vi "Initialize.vi"(7 "Serial Configuration":T1={"Baud Rate"=9600, "Parity"=0, "Data Bits"=7, "Stop Bits"=10, "Flow Control"=0} {"Flow Control" items=["None", "XON/XOFF", "RTS/CTS", "XON/XOFF & RTS/CTS", "DTR/DSR", "XON/XOFF & DTR/DSR"]; "Stop Bits" items=["1.0"=10, "1.5"=15, "2.0"=20]; "Data Bits" items=["7"=7, "8"=8]; "Parity" items=["None", "Odd", "Even", "Mark", "Space"]; "Baud Rate" items=["300"=300, "600"=600, "1200"=1200, "2400"=2400, "4800"=4800, "9600"=9600, "19200"=19200]}, 8 "error in (no error)":errorcluster, 9 "Reset (True)":bool=TRUE, 10 "ID Query (True)":bool=TRUE, 11 "VISA resource name":refnum<visa-resource-name>) -> (0 "error out":errorcluster, 3 "VISA resource name out":refnum<visa-resource-name>)   [LabVIEW 2019]
doc: "Establishes communication with the instrument and optionally performs an instrument identification query and/or an instrument reset. It also places the instrument in a default state needed for other instrument driver operations. Therefore, call this VI before calling other instrument driver VIs for this instrument. Generally, you need to call the <b>Initialize</b> VI only once at the beginning of an application."
uses:
  <instrlib>/Faulhaber RS232/Faulhaber RS232.lvlib
panel:
  # "(c) 2014 <Enter Company Name Here>.  ALL RIGHTS RESERVED."
  # "EDIT: Change control description to remove example text for buses not supported."
  # "EDIT: Serial settings must match those on the physical instrument.  Review user's manual to determine the correct Flow Control protocol for the instrument.  \"None\" is the least robust option for this setting, and could lead to unreliable data transmission."
  # "EDIT: If your instrument does not support ID query or Reset, remove the ID Query or Reset control from the front panel and delete the case structure with the ID Query or Reset code from the block diagram."
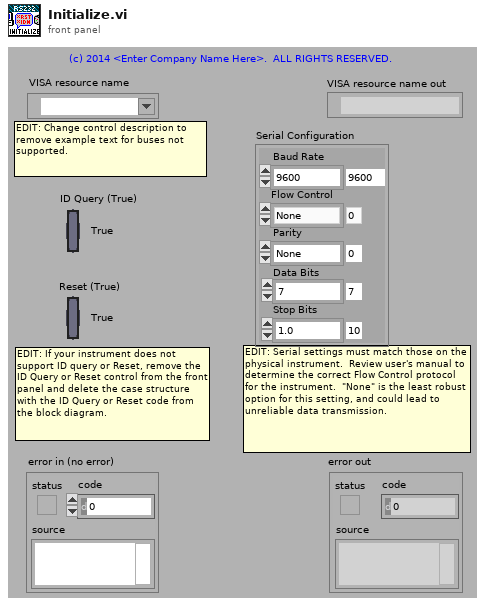
[diagram p1: front panel]
types:
  T1 = cluster{"Baud Rate":u32, "Parity":u16, "Data Bits":u16, "Stop Bits":u16, "Flow Control":u16}
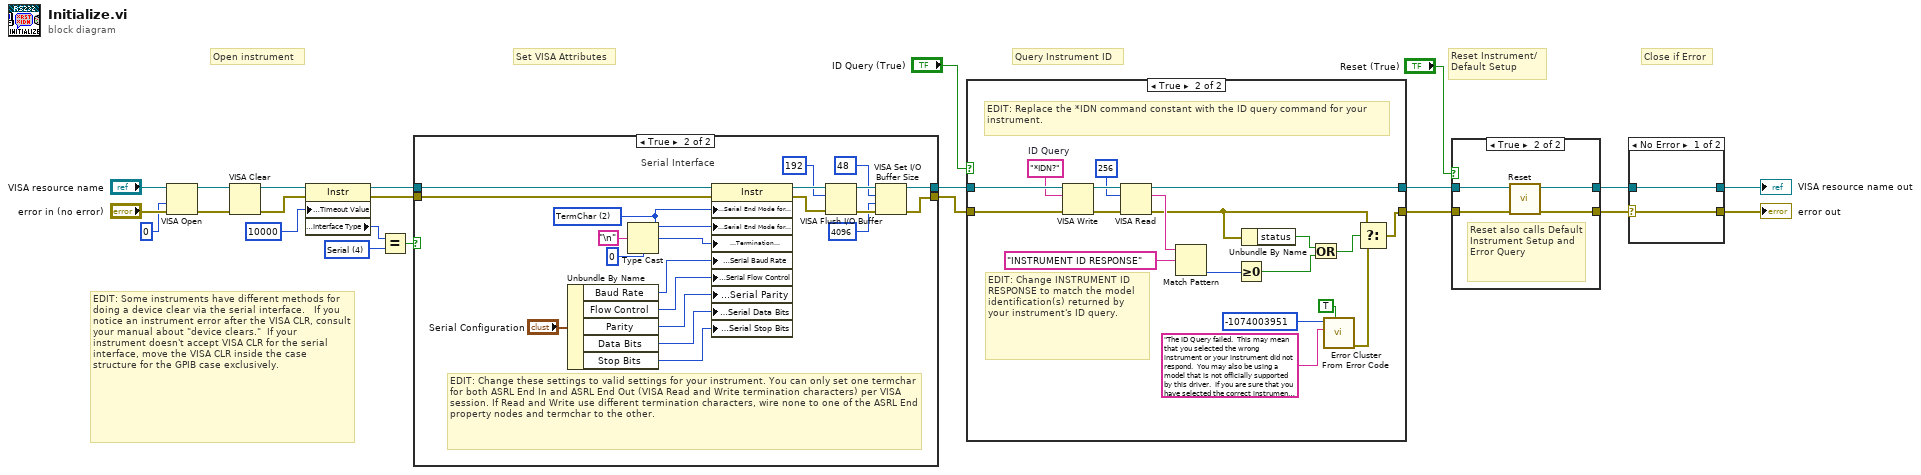
[diagram p0: block diagram]
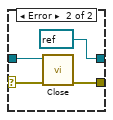
[diagram p3: hidden frame]
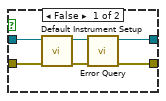
[diagram p4: hidden frame]
diagram:
  w10 = u16 4 items=["GPIB"=1, "VXI"=2, "GPIB-VXI"=3, "Serial"=4, "PXI"=5, "TCPIP"=6, "USB"=7] ("Interface Information:Interface Type")
  # "EDIT: Some instruments have different methods for doing a device clear via the serial interface.   If you notice an instrument error after the VISA CLR, consult your manual about \"device clears.\"  If your instrument doesn't accept VISA CLR for the serial interface, move the VISA CLR inside the case  structure for the GPIB case exclusively."
  # "Set VISA Attributes"
  # "Close if Error"
  # "Query Instrument ID"
  # "Reset Instrument/\nDefault Setup"
  # "Open instrument"
  n1 = VISA Open(access mode=u32 0, error in (no error)="error in (no error)", VISA resource name="VISA resource name") -> (VISA resource name=w8:refnum<visa-resource-name>, error out=w7:errorcluster)  [unwired: 2 in]
  n2 = VISA Clear(VISA resource name=w8, error in (no error)=w7) -> (VISA resource name out=w6:refnum<visa-resource-name>, error out=w5:errorcluster)
  n3 = property class="Instr"(reference=w6, error in=w5, "General Settings:Timeout Value"=u32 10000) -> (reference out=w13:refnum<visa-resource-name>, error out=w12:errorcluster, "Interface Information:Interface Type"=w17:u16)
  n4 = Equal?(x=w17, y=w10) -> (x = y?=w11:bool)
  n5 = case shown="True" w11 {
    tunnel: [w24 w43] -> w15
    tunnel: [w25 w40] -> w14
    tunnel: w13 -> [w24 w45]
    tunnel: w12 -> [w25 w46]
    frame False {
      # "EDIT: Remove interfaces not supported by your instrument."
      # "GPIB, TCP/IP, and USB Interface"
    }
    frame True {
      w33 = u16 2 items=["None", "LastBit", "TermChar"] ("Serial Settings:Serial End Mode for Reads")
      # "EDIT: Change these settings to valid settings for your instrument. You can only set one termchar for both ASRL End In and ASRL End Out (VISA Read and Write termination characters) per VISA session. If Read and Write use different termination characters, wire none to one of the ASRL End property nodes and termchar to the other."
      # "Serial Interface"
      n6 = Unbundle By Name("Serial Configuration") -> ("Baud Rate"=w31:u32, "Flow Control"=w27:u16, "Parity"=w29:u16, "Data Bits"=w30:u16, "Stop Bits"=w26:u16)
      n7 = Type Cast(type=u8 0, x="\n" ("Line Feed Constant")) -> (*(type *) &x=w32:u8)
      n8 = property class="Instr"(reference=w45, error in=w46, "Serial Settings:Serial End Mode for Reads"=w33, "Serial Settings:Serial End Mode for Writes"=w33, "Message Based Settings:Termination Character"=w32, "Serial Settings:Serial Baud Rate"=w31, "Serial Settings:Serial Flow Control"=w27, "Serial Settings:Serial Parity"=w29, "Serial Settings:Serial Data Bits"=w30, "Serial Settings:Serial Stop Bits"=w26) -> (reference out=w39:refnum<visa-resource-name>, error out=w42:errorcluster)
      n9 = VISA Flush I/O Buffer(VISA resource name=w39, mask (16)=u16 192, error in (no error)=w42) -> (VISA resource name out=w44:refnum<visa-resource-name>, error out=w41:errorcluster)
      n10 = VISA Set I/O Buffer Size(VISA resource name=w44, mask (16)=u16 48, size (4096)=u32 4096 ("size (0)"), error in (no error)=w41) -> (VISA resource name out=w43:refnum<visa-resource-name>, error out=w40:errorcluster)
    }
  }
  n11 = case shown="True" "ID Query (True)" {
    tunnel: [w47 w67] -> w22
    tunnel: [w48 w64] -> w23
    tunnel: w15 -> [w48 w65]
    tunnel: w14 -> [w47 w66]
    frame False {
    }
    frame True {
      w58 = "*IDN?"  # ID Query
      # "EDIT: Replace the *IDN command constant with the ID query command for your instrument."
      # "EDIT: Change INSTRUMENT ID RESPONSE to match the model identification(s) returned by your instrument's ID query."
      n12 = VISA Write(VISA resource name=w65, write buffer=w58, error in (no error)=w66) -> (VISA resource name out=w62:refnum<visa-resource-name>, error out=w61:errorcluster)  [unwired: 1 out]
      n13 = VISA Read(VISA resource name=w62, byte count=u32 256, error in (no error)=w61) -> (VISA resource name out=w64:refnum<visa-resource-name>, read buffer=w63:string, error out=w52:errorcluster)  [unwired: 1 out]
      n14 = Match Pattern(string=w63, regular expression="INSTRUMENT ID RESPONSE") -> (offset past match=w53:i32)  [unwired: 1 in, 3 out]
      n15 = Greater Or Equal To 0?(x=w53) -> (x >= 0?=w50:bool)
      n16 = Unbundle By Name(w52) -> ("status"=w51:bool)
      n17 = Or(x=w51, y=w50) -> (x .or. y?=w49:bool)
      n18 = call <vilib>:"Error Cluster From Error Code.vi"("show call chain? (False)"=TRUE, "error message (\"\")"="The ID Query failed.  This may mean that you selected the wrong instrument or your instrument did not respond.  You may also be using a model that is not officially supported by this driver.  If you are sure that you have selected the correct instrument and it is responding, try disabling the ID Query." ("Source (VI Name)"), "error code (0)"=-1074003951 ("Code")) -> ("error out"=w57:errorcluster)  [unwired: 6 in]
      n19 = Select(t=w52, s=w49, f=w57) -> (s? t:f=w67:errorcluster)
    }
  }
  n20 = case shown="True" "Reset (True)" {
    tunnel: w22 -> [w72 w74]
    tunnel: [w69 w77] -> w1
    tunnel: w23 -> [w73 w75]
    tunnel: [w70 w76] -> w2
    frame False {
      n21 = call <instrlib>:"Default Instrument Setup.vi"("error in (no error)"=w72, "VISA resource name"=w73) -> ("error out"=w68:errorcluster, "VISA resource name out"=w71:refnum<visa-resource-name>)  [unwired: 8 in]
      n22 = call <instrlib>:"Error Query.vi"("error in (no error)"=w68, "VISA resource name"=w71) -> ("error out"=w69:errorcluster, "VISA resource name out"=w70:refnum<visa-resource-name>)  [unwired: 6 in, 2 out]
    }
    frame True {
      # "Reset also calls Default Instrument Setup and Error Query"
      n23 = call <instrlib>:"Reset.vi"("error in (no error)"=w74, "VISA resource name"=w75) -> ("error out"=w77:errorcluster, "VISA resource name out"=w76:refnum<visa-resource-name>)  [unwired: 8 in]
    }
  }
  n24 = case shown="No Error" w1 {
    selector: w1 -> [w78 w81]
    tunnel: w2 -> [w79 w82]
    tunnel: [w79 refnum<visa-resource-name> refnum ("VISA resource name out")] -> w4
    tunnel: [w78 w83] -> w3
    frame No Error {
    }
    frame Error {
      n25 = call <instrlib>:"Close.vi"("error in (no error)"=w81, "VISA resource name"=w82) -> ("error out"=w83:errorcluster)  [unwired: 9 in]
    }
  }
  "VISA resource name out" <- w4
  "error out" <- w3
